vi "CalculateTimes.vi"(8 "error in":errorcluster, 9 "Number of Dymin Steps":u8=1 min=1 max=4 step=1, 10 "Dwell Time (us)":dbl, 11 "Time (us)":dbl[](array[numeric])=[0.0, 0.0, 0.0, 0.0] min=0.0 max=10000.0 step=0.0125) -> (0 "error out":errorcluster, 1 "Dwell Time (bits)":u32, 2 "Time (bits)":u32[](array[numeric]), 3 "Time (us)":dbl[](array[numeric]) min=0.0 max=1.0, 5 "Times Bad?":bool)   [LabVIEW 2016]
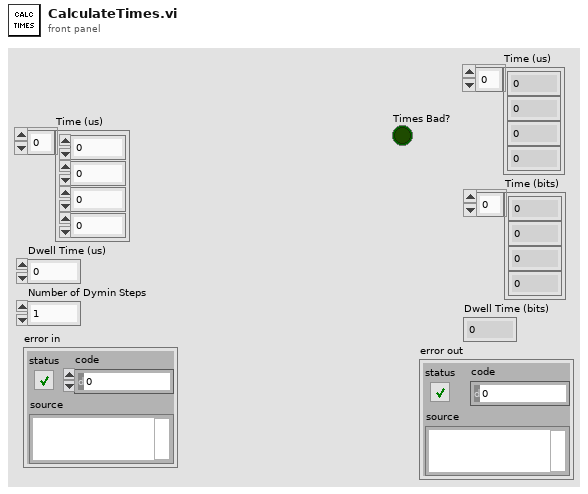
[diagram p1: front panel]
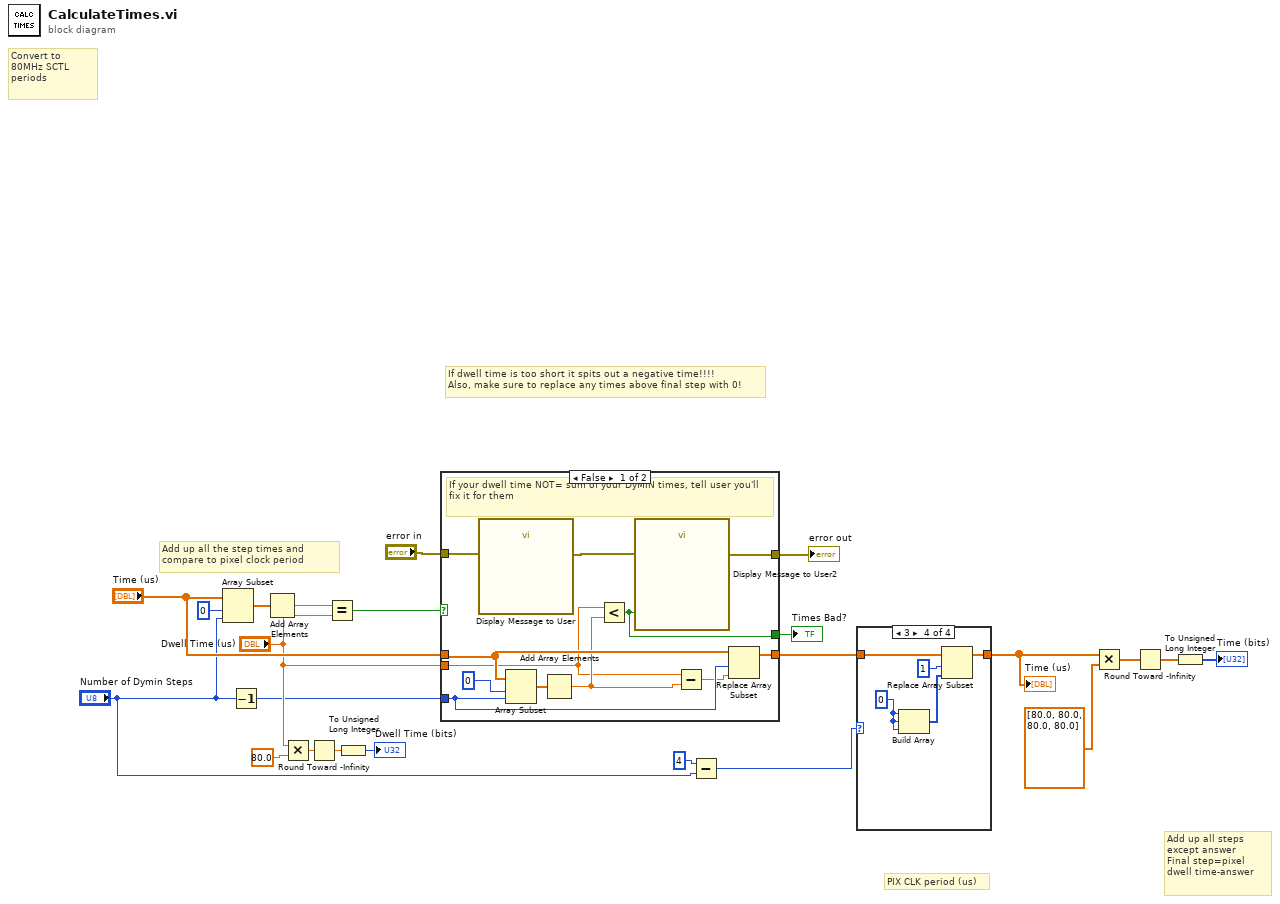
[diagram p0: block diagram]
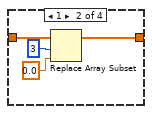
[diagram p3: hidden frame]
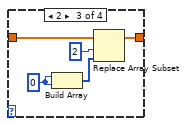
[diagram p4: hidden frame]
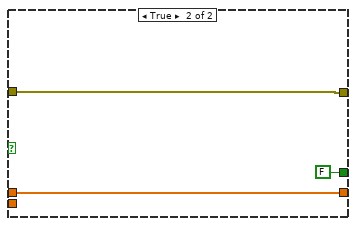
[diagram p5: hidden frame]
diagram:
  # "If dwell time is too short it spits out a negative time!!!!\nAlso, make sure to replace any times above final step with 0!"
  # "Add up all the step times and compare to pixel clock period"
  # "Add up all steps except answer\nFinal step=pixel dwell time-answer"
  # "PIX CLK period (us)"
  # "Convert to 80MHz SCTL periods"
  n1 = Array Subset(array="Time (us)", index=u8 0, length="Number of Dymin Steps") -> (w8:dbl[])
  n2 = Decrement(x="Number of Dymin Steps") -> (x-1=w7:u8)
  n3 = Add Array Elements(numeric array=w8) -> (sum=w6:dbl)
  n4 = Multiply(x="Dwell Time (us)", y=80.0) -> (x*y=w15:dbl)
  n5 = Round Toward -Infinity(1:w15) -> (0:w14:dbl)
  n6 = Equal?(x=w6, y="Dwell Time (us)") -> (x = y?=w5:bool)
  n7 = To Unsigned Long Integer(number=w14) -> (unsigned 32bit integer=→"Dwell Time (bits)":u32)
  n8 = case shown="False" w5 {
    tunnel: "Time (us)" -> [w29 w37]
    tunnel: [w30 w37] -> w2
    tunnel: w7 -> [w33 _]
    tunnel: "error in" -> [w35 w38]
    tunnel: [w25 w38] -> w10
    tunnel: "Dwell Time (us)" -> [w27 _]
    tunnel: [w24 FALSE] -> w1
    frame False {
      # "If your dwell time NOT= sum of your DyMIN times, tell user you'll fix it for them"
      n9 = call "Display Message to User"("error in (no error)"=w35) -> ("error out"=w26:errorcluster)  [unwired: 9 in, 1 out]
      n10 = Array Subset(array=w29, index=u8 0, length=w33) -> (w32:dbl[])
      n11 = Add Array Elements(numeric array=w32) -> (sum=w28:dbl)
      n12 = Less?(x=w27, y=w28) -> (x < y?=w24:bool)
      n13 = call "Display Message to User2"("error in (no error)"=w26, "Enable"=w24) -> ("error out"=w25:errorcluster)  [unwired: 8 in, 1 out]
      n14 = Subtract(x=w27, y=w28) -> (x-y=w31:dbl)
      n15 = Replace Array Subset(array=w29, new element=w31, index=w33) -> (w30:dbl[])
    }
    frame True {
    }
  }
  "error out" <- w10
  "Times Bad?" <- w1
  n16 = Subtract(x=u8 4, y="Number of Dymin Steps") -> (x-y=w3:u8)
  n17 = case shown="3" w3 {
    tunnel: [w39 w42 w45 w51] -> w18
    tunnel: w2 -> [w39 w40 w44 w49]
    frame 0, Default {
    }
    frame 1 {
      n18 = Replace Array Subset(array=w40, new element=0.0 ("element"), index=u8 3) -> (w42:dbl[])
    }
    frame 2 {
      w48 = u8 0 ("element")
      n19 = Build Array(w48, w48) -> (w47:u8[])
      n20 = Replace Array Subset(array=w44, new element=w47, index=u8 2) -> (w45:dbl[])
    }
    frame 3 {
      w50 = 0 ("element")
      n21 = Build Array(w50, w50, w50) -> (w53:i32[])
      n22 = Replace Array Subset(array=w49, new element=w53, index=1) -> (w51:dbl[])
    }
  }
  "Time (us)" <- w18
  n23 = Multiply(x=w18, y=dbl[] [80.0, 80.0, 80.0, 80.0]) -> (x*y=w22:dbl[])
  n24 = Round Toward -Infinity(1:w22) -> (0:w21:dbl[])
  n25 = To Unsigned Long Integer(number=w21) -> (unsigned 32bit integer=→"Time (bits)":u32[])
